vi "Close Track.vi"(8 "Error In":errorcluster, 11 "Track (File) References":T1) -> (0 "Error Out":errorcluster)   [LabVIEW 2014]
doc: "Close all 4 track files references."
uses:
  Controls/Track (File) References.ctl
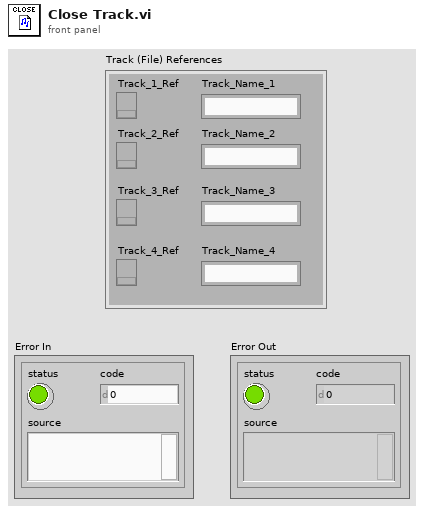
[diagram p1: front panel]
types:
  T1 = typedef "Track (File) References.ctl" = cluster{"Track_1_Ref":refnum<k34>, "Track_2_Ref":refnum<k34>, "Track_3_Ref":refnum<k34>, "Track_4_Ref":refnum<k34>, "Track_Name_1":string, "Track_Name_2":string, "Track_Name_3":string, "Track_Name_4":string}
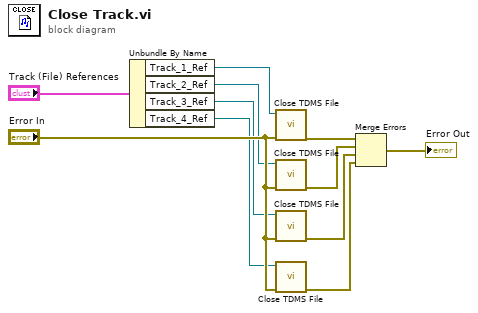
[diagram p0: block diagram]
diagram:
  n1 = Unbundle By Name("Track (File) References") -> ("Track_1_Ref"=w9:refnum<k34>, "Track_2_Ref"=w8:refnum<k34>, "Track_3_Ref"=w7:refnum<k34>, "Track_4_Ref"=w6:refnum<k34>)
  n2 = call "Close TDMS File.vi"("Error In"="Error In", "TDMS Reference In"=w9) -> ("Error Out"=w5:errorcluster)  [unwired: 9 in]
  n3 = call "Close TDMS File.vi"("Error In"="Error In", "TDMS Reference In"=w8) -> ("Error Out"=w4:errorcluster)  [unwired: 9 in]
  n4 = call "Close TDMS File.vi"("Error In"="Error In", "TDMS Reference In"=w7) -> ("Error Out"=w3:errorcluster)  [unwired: 9 in]
  n5 = call "Close TDMS File.vi"("Error In"="Error In", "TDMS Reference In"=w6) -> ("Error Out"=w2:errorcluster)  [unwired: 9 in]
  n6 = Merge Errors(w5, w4, w3, w2) -> (→"Error Out":errorcluster)
